vi "FTW-Test-JSON-NumericParse.vi"() -> ()   [LabVIEW 2015]
uses:
  source/JSON/FTW-JSON-LexicalScan.ctl
panel:
  out "error out":errorcluster
  out "Array 3":errorcluster[](array[cluster])
  out "Array 2":variant[](array[variant])
  in  "Array":string[](array[string])=["1", "1.2", "-1", "-1.2", "1e1", "1e-1", "1.2e3", "1.2e-3"]
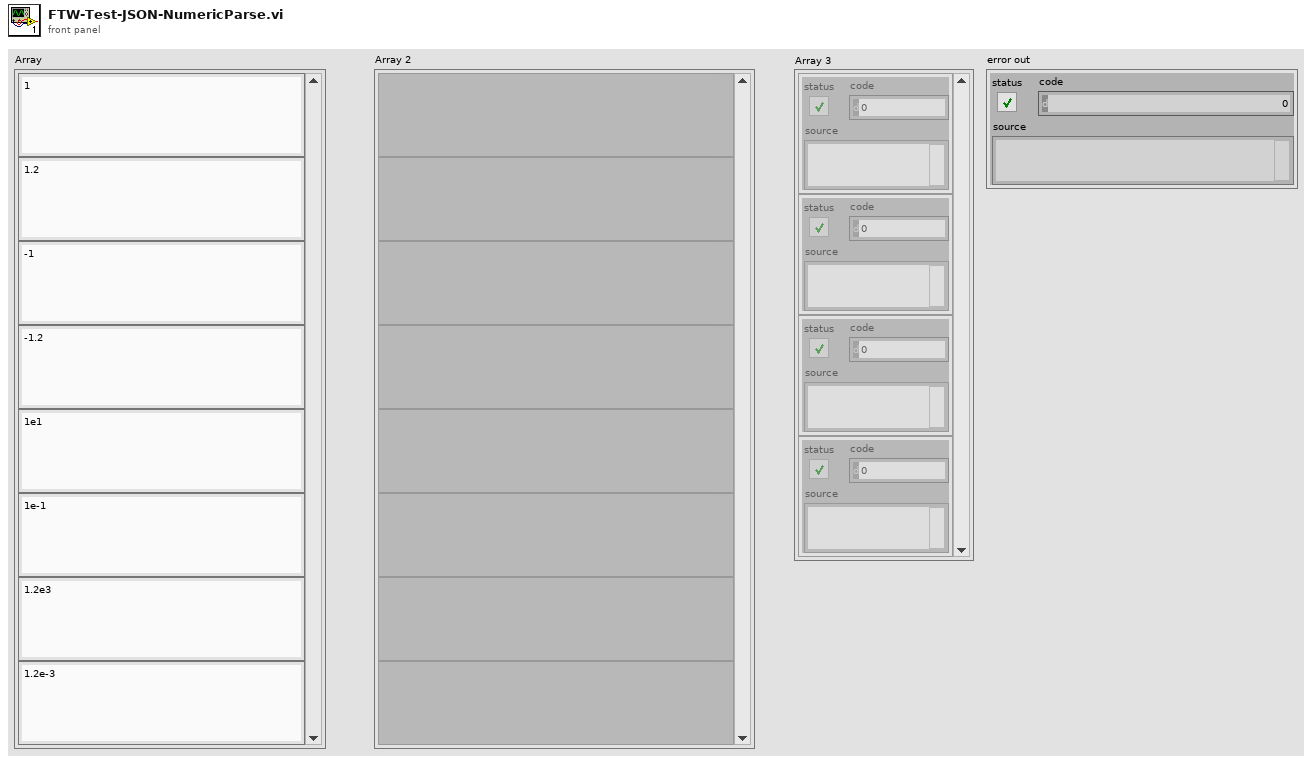
[diagram p1: front panel]
types:
  T1 = typedef "FTW-JSON-LexicalScan.ctl" = cluster{"String":string, "Position":i32, "Line":i32, "Column":i32, "Last Column":i32}
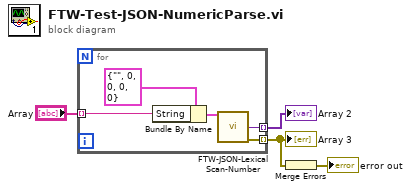
[diagram p0: block diagram]
diagram:
  n1 = for {
    tunnel: "Array" -> [w7] mode=indexing
    tunnel: [w6] -> w3 mode=indexing
    tunnel: [w5] -> w2 mode=indexing
    n2 = Bundle By Name(cluster=T1 {"String"="", "Position"=0, "Line"=0, "Column"=0, "Last Column"=0} ("JSON String"), "String"=w7) -> (w8:T1)
    n3 = call "FTW-JSON-LexicalScan-Number.vi"("JSON String"=w8) -> ("Number"=w6:variant, "error out"=w5:errorcluster)  [unwired: 12 in, 1 out]
  }
  "Array 2" <- w3
  "Array 3" <- w2
  n4 = Merge Errors(w2) -> (→"error out":errorcluster)
